vi "Send Data to UI.vi"(10 "Waveform Data Array":waveform(sgl)[](array[waveform]) caption="波形数组") -> (0 "error out":errorcluster caption="错误输出")   [LabVIEW 2013]
uses:
  Globals/Global - Monitoring Variables.vi
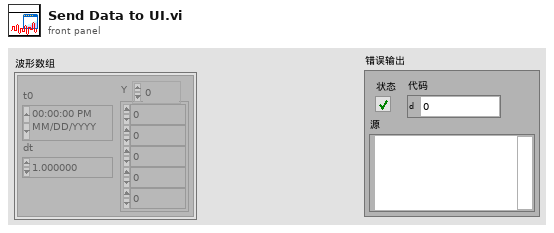
[diagram p1: front panel]
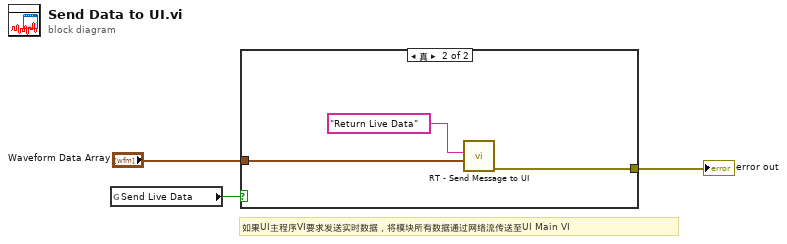
[diagram p0: block diagram]
diagram:
  # "如果UI主程序VI要求发送实时数据，将模块所有数据通过网络流传送至UI Main VI"
  n1 = global read "Global - Monitoring Variables.vi" "Send Live Data"() -> (w3:bool)
  n2 = case shown="真" w3 {
    tunnel: "Waveform Data Array" -> [_ w4]
    tunnel: [_ w6] -> w2
    frame False {
    }
    frame True {
      n3 = call "RT - Send Message to UI.vi"("Message Data"=w4, "Message"="Return Live Data" ("group name in (Untitled)")) -> ("error out"=w6:errorcluster)  [unwired: 9 in]
    }
  }
  "error out" <- w2
